vi "Connect Error wires in Reset Case.vi"(0 "Case Sel Refnum":refnum<vi>, 11 "error in (no error)":errorcluster) -> (4 "Case Sel Refnum Out":refnum<vi>, 15 "error out":errorcluster)   [LabVIEW 2021, in "Migrator.lvlib"]
uses:
  Migrator.lvlib
  Migrator Reusables/Migrator Reusables.lvlib
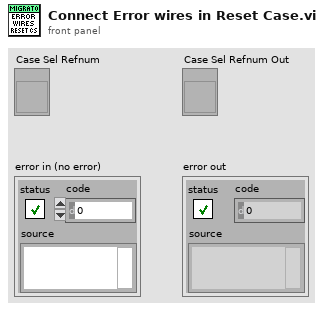
[diagram p1: front panel]
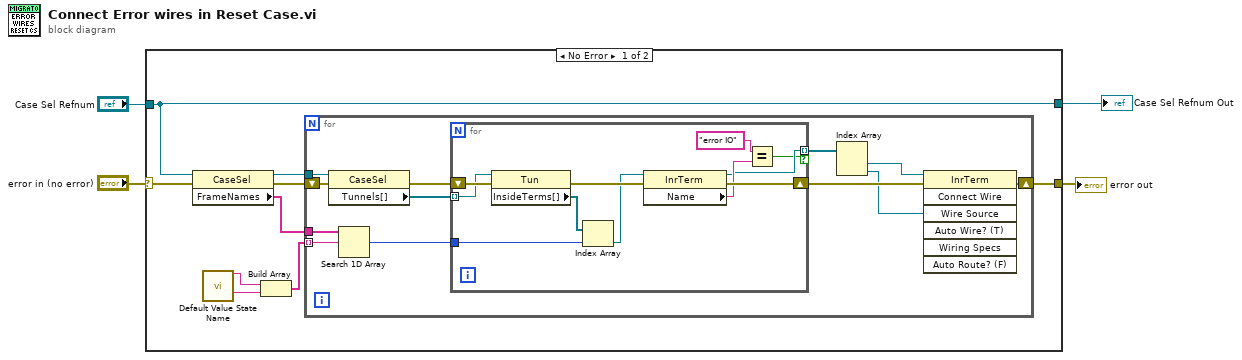
[diagram p0: block diagram]
diagram:
  n1 = case shown="No Error" "error in (no error)" {
    selector: "error in (no error)" -> [w12 w38]
    tunnel: [w9 w38] -> w4
    tunnel: "Case Sel Refnum" -> [w8 w37]
    tunnel: [w8 w37] -> w1
    frame No Error {
      n2 = property class="CaseSel"(reference=w8, error in=w12) -> (reference out=w13:refnum<vi>, error out=w10:errorcluster, "FrameNames"=w11:string[])
      n3 = call "Default Value State Name.vi"() -> ("Set Default Value State"=w7:string, "Load Values"=w6:string)  [unwired: 12 in, 2 out]
      n4 = Build Array(w7, w6) -> (w5:string[])
      n5 = for {
        tunnel: w13 -> [w25]
        tunnel: w11 -> [w24]
        tunnel: w5 -> [w23] mode=indexing
        shift-right: [w19] -> w9
        shift-left: w10 -> [w22]
        n6 = property class="CaseSel"(reference=w25, error in=w22) -> (error out=w21:errorcluster, "Tunnels[]"=w18:refnum<vi>[])  [unwired: 1 out]
        n7 = Search 1D Array(1D array=w24, element=w23) -> (index of element=w17:i32)  [unwired: 1 in]
        n8 = for {
          shift-right: [w34] -> w20
          shift-left: w21 -> [w36]
          tunnel: w18 -> [w30] mode=indexing
          tunnel: w17 -> [w29]
          tunnel: [w27] -> w16 mode=indexing if=w26
          n9 = property class="Tun"(reference=w30, error in=w36) -> (error out=w35:errorcluster, "InsideTerms[]"=w31:refnum<vi>[])  [unwired: 1 out]
          n10 = Index Array(array=w31, index=w29) -> (element=w28:refnum<vi>)
          n11 = property class="InrTerm"(reference=w28, error in=w35) -> (reference out=w27:refnum<vi>, error out=w34:errorcluster, "Name"=w33:string)
          n12 = Equal?(x="error IO" ("y"), y=w33) -> (x = y?=w26:bool)
        }
        n13 = Index Array(array=w16) -> (element #1=w15:refnum<vi>, element #2=w14:refnum<vi>)  [unwired: 2 in]
        n14 = invoke class="InrTerm" method="Connect Wire"(reference=w15, error in=w20, "Wire Source"=w14) -> (error out=w19:errorcluster)  [unwired: 4 in, 6 out]
      }
    }
    frame Error {
    }
  }
  "error out" <- w4
  "Case Sel Refnum Out" <- w1
